vi "Command WPIN.vi"(0 "Serial Devices in":refnum<class "Serial Devices.lvclass">, 1 "Device":string, 5 "Puerto":u8, 7 "Pin":u8, 9 "Valor":string, 11 "error in (no error)":errorcluster) -> (4 "Serial Devices out":refnum<class "Serial Devices.lvclass">, 6 "Command":string, 10 "Expected":string, 15 "error out":errorcluster)   [LabVIEW 2019, in "Serial Devices.lvlib" / "Serial Devices.lvclass"]
uses:
  Serial Devices.lvclass
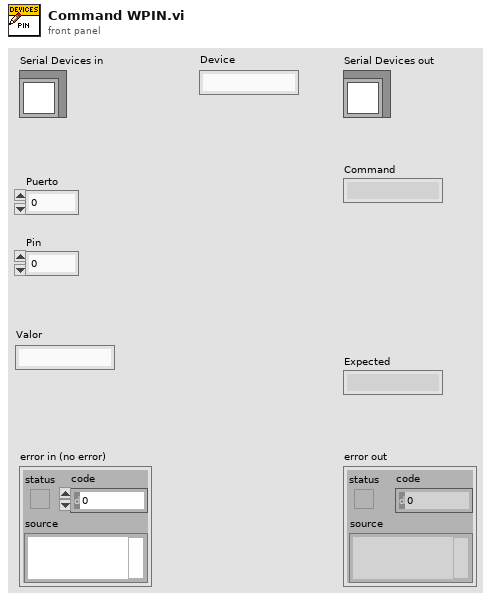
[diagram p1: front panel]
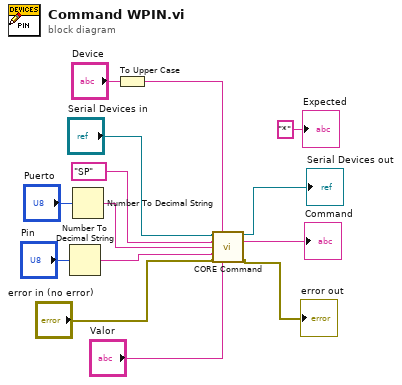
[diagram p0: block diagram]
diagram:
  n1 = Number To Decimal String(number="Pin") -> (decimal integer string=w2:string)  [unwired: 1 in]
  n2 = Number To Decimal String(number="Puerto") -> (decimal integer string=w7:string)  [unwired: 1 in]
  n3 = To Upper Case(1:"Device") -> (0:w6:string)
  n4 = call "CORE Command.vi"("Serial Devices in"="Serial Devices in", "Device"=w6, "Command"="SP", "Chanel-Puerto"=w7, "Param-Pin"=w2, "error in (no error)"="error in (no error)", "Valor"="Valor") -> ("Serial Devices out"=→"Serial Devices out":refnum<class "Serial Devices.lvclass">, "Command"=→"Command":string, "error out"=→"error out":errorcluster)  [unwired: 5 in, 1 out]
  "Expected" <- "*" ("Expected")
